vi "Get ProcessMdFuncName.vi"(11 "ProcessMdFuncName in":string caption="Embedding Model URL in") -> (3 "ProcessMdFuncName out":string)   [LabVIEW 2023, in "LabVIEW RAG.lvlib"]
uses:
  LabVIEW RAG.lvlib
  AI RAG Globals.vi
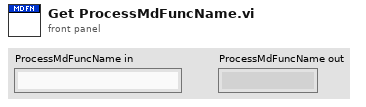
[diagram p1: front panel]
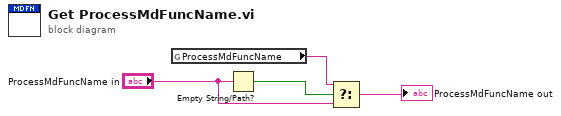
[diagram p0: block diagram]
diagram:
  n1 = global read "AI RAG Globals.vi" "ProcessMdFuncName"() -> (w4:string)
  n2 = Empty String/Path?(string/path="ProcessMdFuncName in") -> (empty?=w3:bool)
  n3 = Select(t=w4, s=w3, f="ProcessMdFuncName in") -> (s? t:f=→"ProcessMdFuncName out":string)
